vi "GUI Final.vi"() -> ()   [LabVIEW 2014]
uses:
  <vilib>/Instr/_visa.llb/VISA Configure Serial Port (Instr).vi
panel:
  out "pass ACK":bool
  out "Threshold sent":bool
  out "no of trials read":bool
  out "PC on Ack":bool
  out "Reset#":i32
  in  "Reset":bool
  out "return count read":u32
  in  "VISA resource name":refnum<visa-resource-name>
  out "Iteration":i32
  in  "Tab Control":enum32{"Page 1", "Page 2", "Page 3"}(tab)
  in  "Password":string
  in  "Threshold":string
  out "read buffer":string
  out "password is wrong":bool
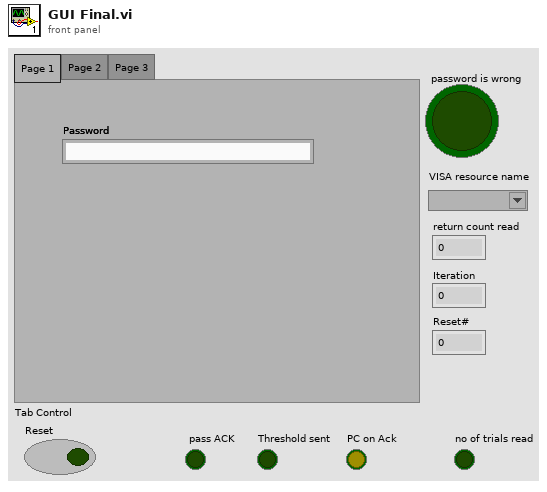
[diagram p1: front panel]
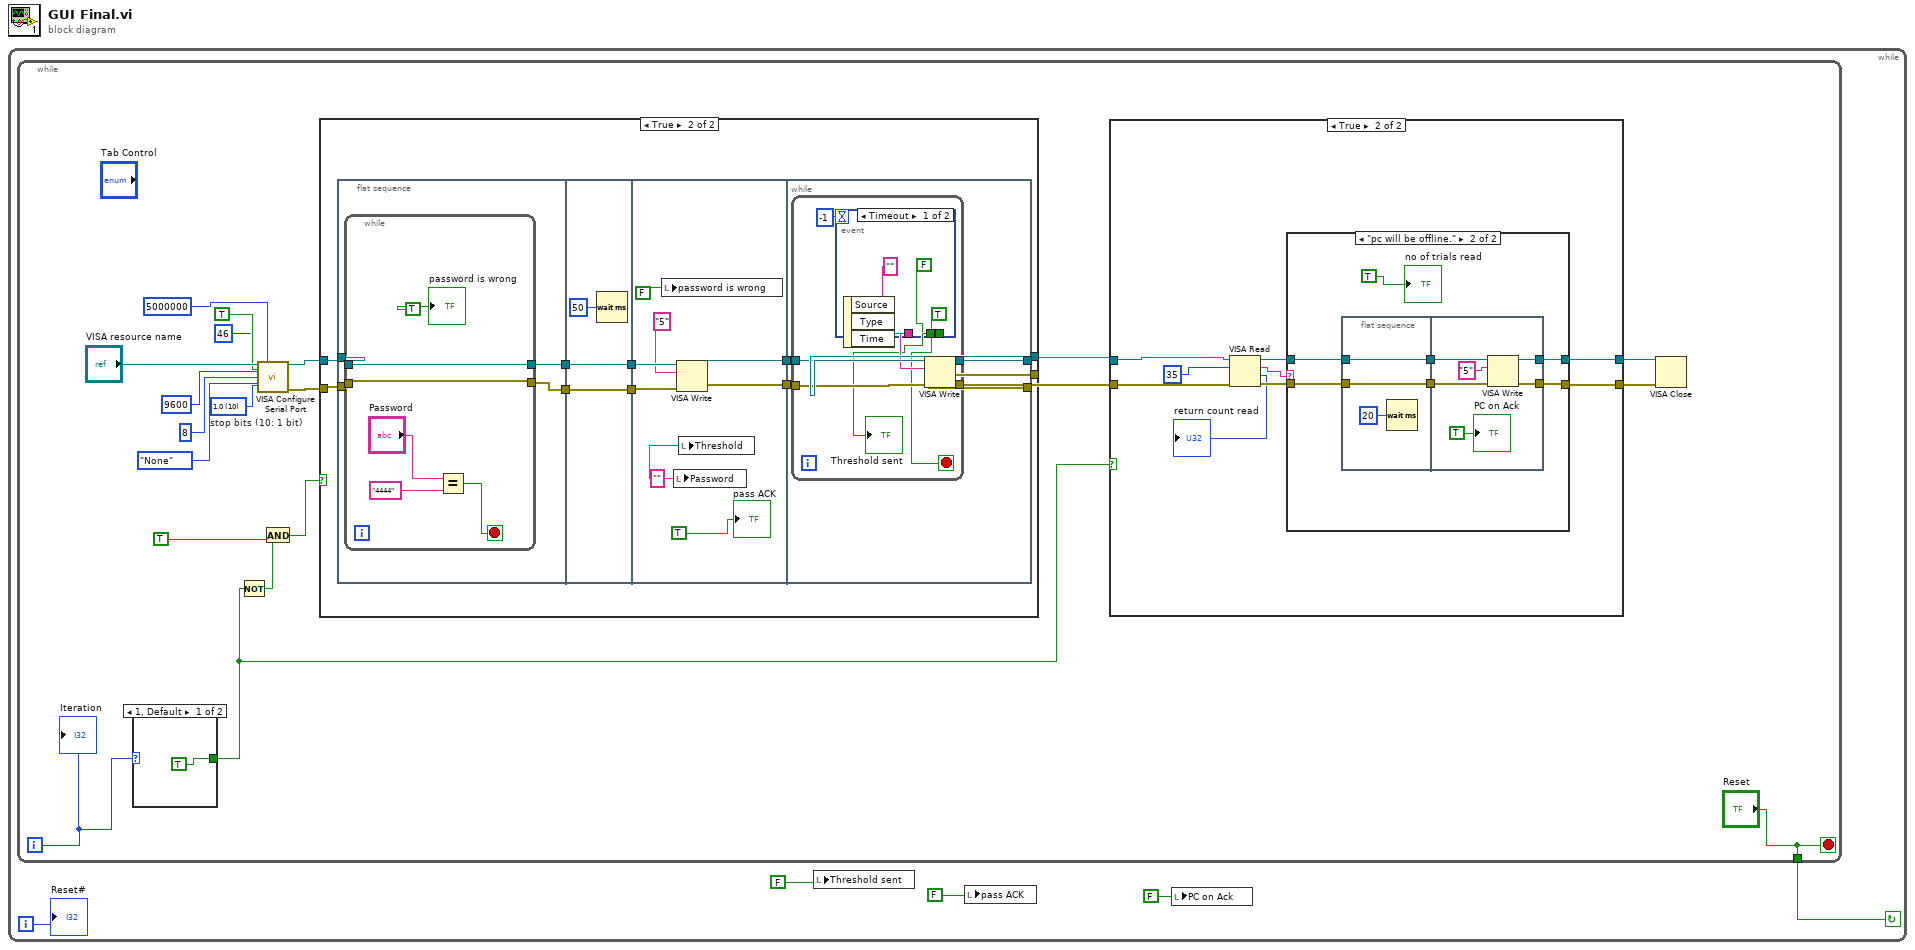
[diagram p0: block diagram]
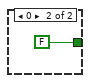
[diagram p2: hidden frame]
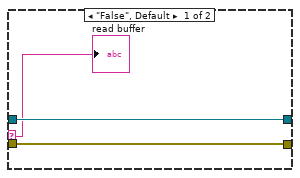
[diagram p4: hidden frame]
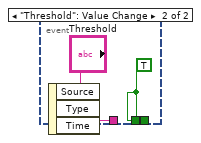
[diagram p6: hidden frame]
diagram:
  n1 = while {
    i -> [w5]
    stop <- w4 continue-if-true
    n2 = while {
      tunnel: ["Reset"] -> w4
      i -> [w9]
      stop <- "Reset" stop-if-true
      w22 = u16 10 items=["1.0"=10, "1.5"=15, "2.0"=20]  # stop bits (10: 1 bit)
      n3 = case shown="1, Default" w9 {
        tunnel: [TRUE FALSE] -> w8
        frame 1, Default {
        }
        frame 0 {
        }
      }
      n4 = Not(x=w8) -> (.not. x?=w17:bool)
      n5 = call-poly "VISA Configure Serial Port"("VISA resource name"="VISA resource name", "timeout (10sec)"=u32 5000000, "termination char\n(0xA = '\\n' = LF)"=u8 46 ("termination char\n(0xA = '\\n' = LF)"), "Enable Termination\nChar (T)"=TRUE ("Enable Termination\nChar (T)"), "baud rate (9600)"=u32 9600, "data bits (8)"=u16 8, "parity (0:none)"=enum16{"None", "Odd", "Even", "Mark", "Space"}."None", "stop bits (10: 1 bit)"=w22) -> ("VISA resource name out"=w16:refnum<visa-resource-name>, "error out"=w15:errorcluster)  [unwired: 6 in]
      n6 = And(x=w17, y=TRUE) -> (x .and. y?=w14:bool)
      n7 = case shown="True" w14 {
        tunnel: w15 -> [w59 w69]
        tunnel: [w58 w67] -> w13
        tunnel: [w59 w66] -> w11
        tunnel: w16 -> [w58 w68]
        frame False {
        }
        frame True {
          n8 = flat-sequence {
            tunnel: w69 -> [w73]
            tunnel: w68 -> [w72]
            tunnel: [w71] -> w63
            tunnel: [w70] -> w61
            tunnel: w63 -> [w82]
            tunnel: [w82] -> w62
            tunnel: w61 -> [w81]
            tunnel: [w81] -> w60
            tunnel: w62 -> [w90]
            tunnel: w60 -> [w89]
            tunnel: [w88] -> w65
            tunnel: [w87] -> w64
            tunnel: [w93] -> w67
            tunnel: [w92] -> w66
            tunnel: w65 -> [w94]
            tunnel: w64 -> [w91]
            frame #0 {
              n9 = while {
                tunnel: w73 -> [w78]
                tunnel: w72 -> [w77]
                tunnel: [w78] -> w71
                tunnel: [w77] -> w70
                stop <- w79 stop-if-true
                n10 = Equal?(x="Password", y="4444") -> (x = y?=w79:bool)
                "password is wrong" <- TRUE
              }
            }
            frame #1 {
              n11 = Wait (ms)(milliseconds to wait=u32 50) -> ()  [unwired: 1 out]
            }
            frame #2 {
              w84 = "" ("Password")
              n12 = local write "password is wrong"(FALSE) -> ()
              n13 = local write "Password"(w84) -> ()
              n14 = VISA Write(VISA resource name=w89, write buffer="5", error in (no error)=w90) -> (VISA resource name out=w88:refnum<visa-resource-name>, error out=w87:errorcluster)  [unwired: 1 out]
              n15 = local write "Threshold"(w84) -> ()
              "pass ACK" <- TRUE ("Pass Ack")
            }
            frame #3 {
              n16 = while {
                tunnel: w94 -> [w102]
                tunnel: [w101] -> w93
                tunnel: [w100] -> w92
                tunnel: w91 -> [w99]
                stop <- w96 stop-if-true
                n17 = event shown="[0] Timeout" {
                  selector: _ -> [_ _]
                  dyn-events: _ -> [_ _]
                  timeout: -1 -> [_ _]
                  tunnel: [TRUE w106] -> w96
                  tunnel: ["" "Threshold"] -> w98
                  tunnel: [FALSE w106] -> w95
                  event Timeout {
                    n18 = event-data() -> ()  [unwired: 1 in, 3 out]
                  }
                  event "Threshold": Value Change {
                    w106 = TRUE
                    n19 = event-data() -> ()  [unwired: 1 in, 3 out]
                  }
                }
                "Threshold sent" <- w95
                n20 = VISA Write(VISA resource name=w102, write buffer=w98, error in (no error)=w99) -> (VISA resource name out=w101:refnum<visa-resource-name>, error out=w100:errorcluster)  [unwired: 1 out]
              }
            }
          }
        }
      }
      n21 = case shown="True" w8 {
        tunnel: [w29 w37] -> w12
        tunnel: [w28 w38] -> w10
        tunnel: w13 -> [w29 w32]
        tunnel: w11 -> [w28 w31]
        frame False {
        }
        frame True {
          n22 = VISA Read(VISA resource name=w32, byte count=u32 35, error in (no error)=w31) -> (VISA resource name out=w35:refnum<visa-resource-name>, read buffer=w33:string, return count=→"return count read":u32, error out=w36:errorcluster)
          n23 = case shown="\"pc will be offline.\"" w33 {
            selector: w33 -> [w39 _]
            tunnel: [w40 w45] -> w38
            tunnel: [w41 w46] -> w37
            tunnel: w36 -> [w40 w47]
            tunnel: w35 -> [w41 w48]
            frame "False", Default {
              "read buffer" <- w39
            }
            frame "pc will be offline." {
              n24 = flat-sequence {
                tunnel: w47 -> [w50]
                tunnel: w48 -> [w51]
                tunnel: [w51] -> w44
                tunnel: [w50] -> w43
                tunnel: [w55] -> w46
                tunnel: [w54] -> w45
                tunnel: w44 -> [w57]
                tunnel: w43 -> [w56]
                frame #0 {
                  n25 = Wait (ms)(milliseconds to wait=u32 20) -> ()  [unwired: 1 out]
                }
                frame #1 {
                  n26 = VISA Write(VISA resource name=w57, write buffer="5", error in (no error)=w56) -> (VISA resource name out=w55:refnum<visa-resource-name>, error out=w54:errorcluster)  [unwired: 1 out]
                  "PC on Ack" <- TRUE ("PC on Ack")
                }
              }
              "no of trials read" <- TRUE ("PC on Ack")
            }
          }
        }
      }
      n27 = VISA Close(VISA resource name=w12, error in (no error)=w10) -> ()  [unwired: 1 out]
      "Iteration" <- w9
    }
    n28 = local write "Threshold sent"(FALSE) -> ()
    n29 = local write "pass ACK"(FALSE ("Pass Ack")) -> ()
    n30 = local write "PC on Ack"(FALSE) -> ()
    "Reset#" <- w5
  }
